vi "AI_StreamingAI_MultipleChannels v6.vi"() -> ()   [LabVIEW 2013]
uses:
  <vilib>/Platform/TimedLoop/XDataNode/timing_clust.ctl
  <vilib>/Platform/TimedLoop/XDataNode/nitl_modes.ctl
  <vilib>/Platform/TimedLoop/XDataNode/wakeup.ctl
  <userlib>/DAQNavi Polymorphic VI/create/DAQNavi Create Channel(AI-Voltage).vi
  <userlib>/DAQNavi Polymorphic VI/configure/timing/DAQNavi Timing(Convert Clock).vi
  <userlib>/DAQNavi Polymorphic VI/configure/DAQNavi Get Property/AI/DAQNaviGet_AI_ConvertClock_Rate.vi
  <userlib>/DAQNavi Polymorphic VI/read/DAQNavi Read (Analog 1D Wfm NChan NSamp).vi
  <vilib>/platform/TimedLoop/XDataNode/XDataNode.xnode
  <vilib>/Platform/TimedLoop/XDataNode/XDNodeRunTimeDep.lvlib
panel:
  out "loop time":dbl format="%.6g"
  in  "Read AtoD":bool
  in  "DO":bool[](array[boolean])
  out "Task5":i32
  out "Test":timestamp
  out "Start":timestamp
  out "loops":bool
  out "error out":errorcluster
  out "Waveform Graph":waveform(dbl)[](graph)
  out "value range":string="+/- 5 V" caption="property value"
  out "physical channels":string="DemoDevice,BID#0/ai0:1" caption="property value"
  in  "Samples":u32=1000
  in  "samples per channel":i32=1024
  out "actual convert rate":dbl
  in  "convert clock rate":dbl=1000.0
  in  "stop":bool
  # "Please modify physical channels and value range in Channel Parameters\nthrough DAQNavi Property Assistant VI  in block diagram."
  # "Channel Parameters"
  # "Timing Parameters"
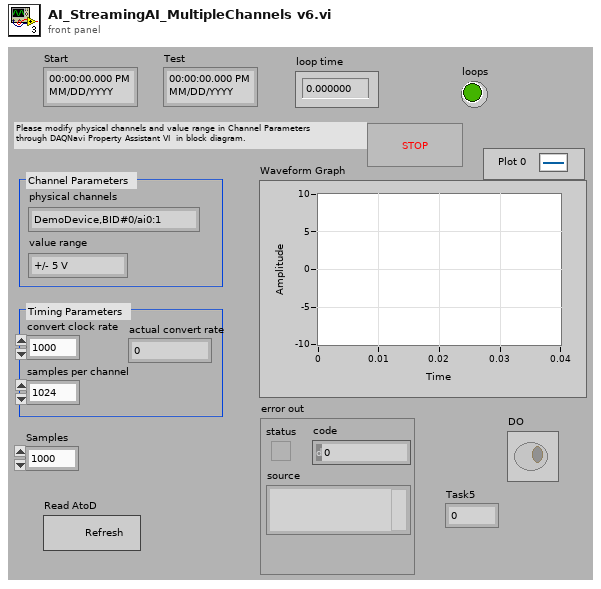
[diagram p1: front panel]
types:
  T1 = typedef "XDNodeRunTimeDep.lvlib/timing_clust.ctl" = cluster{"Expected End [f-1]":u64, "Actual End [f-1]":u64, "Finished Late? [f-1]":bool, "Expected End [i-1]":u64, "Actual End [i-1]":u64, "Finished Late? [i-1]":bool, "Expected Start [i]":u64, "Actual Start [i]":u64, "Expected Start [f]":u64, "Actual Start [f]":u64, "Source Name":string, "Structure Name":string, "Period":i64, "Deadline":i64, "Offset":i64, "Start":i64, "Priority":i32, "Timeout":i32, "Mode":T2, "Wakeup Reason":T3, "Error":errorcluster, "Source Type":string, "Secondary Source Type":string, "Global End Time":u64, "Global Start Time":u64, "Frame Duration":u64, "Iteration Duration":u64, "Assigned CPU":i32, "I/O Scan Engine Mode":u32}
  T2 = typedef "XDNodeRunTimeDep.lvlib/nitl_modes.ctl" = enum32{"No Change", "Process missed periods, maintain original phase", "Discard missed periods, maintain original phase", "Process missed periods, ignore original phase", "Discard missed periods, ignore original phase"}
  T3 = typedef "XDNodeRunTimeDep.lvlib/wakeup.ctl" = enum32{"Normal", "Aborted", "Asynchronous wakeup", "Timing source error", "Timed loop error", "Timeout"}
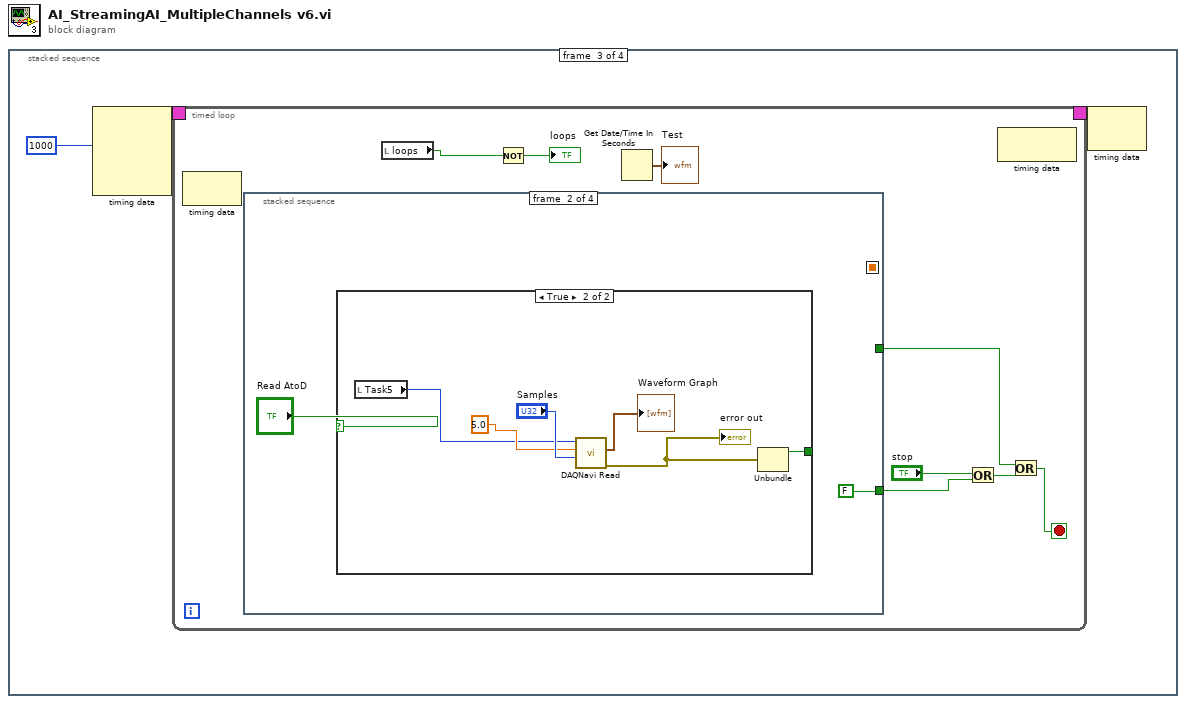
[diagram p0: block diagram]
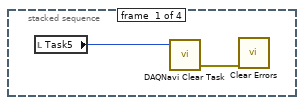
[diagram p2: hidden frame]
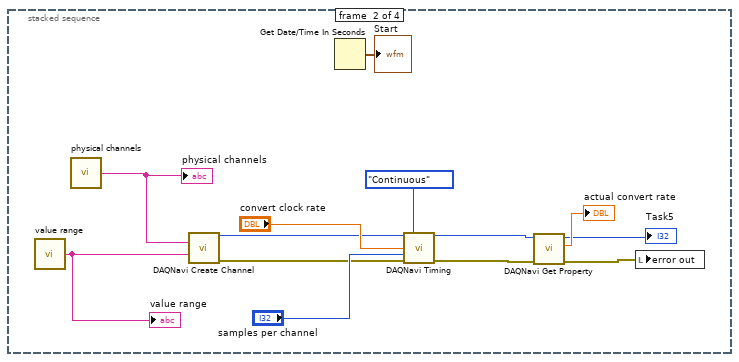
[diagram p3: hidden frame]
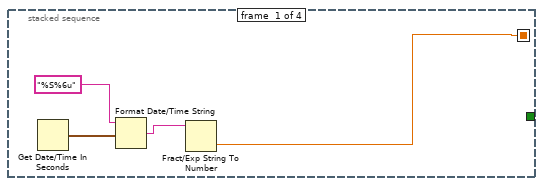
[diagram p4: hidden frame]
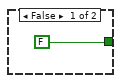
[diagram p5: hidden frame]
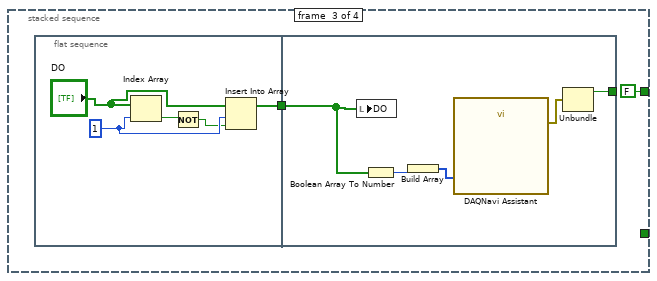
[diagram p6: hidden frame]
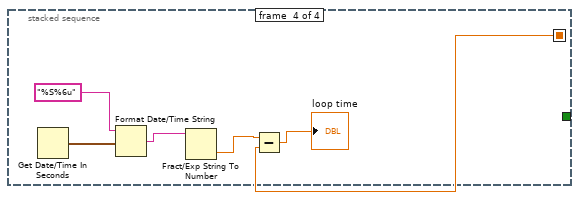
[diagram p7: hidden frame]
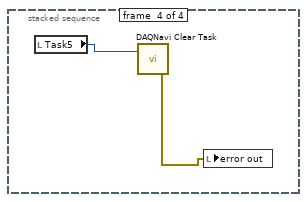
[diagram p8: hidden frame]
diagram:
  n1 = stacked-sequence {
    frame #0 {
      n2 = local read "Task5"() -> (w2:i32)
      n3 = call <userlib>:"DAQNavi Clear Task.vi"("task in"=w2) -> ("error out"=w1:errorcluster)  [unwired: 2 in]
      n4 = call <vilib>:"Clear Errors.vi"("error in (no error)"=w1) -> ()  [unwired: 6 in, 1 out]
    }
    frame #1 {
      n5 = call "value range"() -> ("property value"=w14:string)  [unwired: 1 out]
      "value range" <- w14
      n6 = call "physical channels"() -> ("property value"=w13:string)  [unwired: 1 out]
      "physical channels" <- w13
      n7 = call-poly <userlib>:"DAQNavi Create Channel.vi"("physical channels"=w13, "value range"=w14) -> ("task out"=w5:i32, "error out"=w6:errorcluster)  [unwired: 3 in, 9 out]
      n8 = Get Date/Time In Seconds() -> (seconds since 1Jan1904=→"Start":timestamp)
      n9 = call-poly <userlib>:"DAQNavi Timing.vi"("task in"=w5, "sample mode"=enum16{"Finite", "Continuous"}."Continuous", "rate"="convert clock rate", "samples per channel"="samples per channel", "error in (no error)"=w6) -> ("task out"=w9:i32, "error out"=w10:errorcluster)  [unwired: 1 in, 8 out]
      n10 = call-poly <userlib>:"DAQNavi Get Property.vi"("error in (no error)"=w10, "task in"=w9) -> ("error out"=w4:errorcluster, "rate"=→"actual convert rate":dbl, "task out"=→"Task5":i32)  [unwired: 7 out]
      n11 = local write "error out"(w4) -> ()
    }
    frame #2 {
      n12 = node-c288(1000) -> (w18:T1)  [unwired: 3 in]
      n13 = timed-loop {
        timing: w18 -> [_]
        timing-out: [_] -> w17
        stop <- w23 stop-if-true
        n14 = node-c288() -> ()  [unwired: 1 in, 1 out]
        n15 = stacked-sequence {
          seq-local: [w27 _ _ _] -> [_ _ _ w52]
          tunnel: [_ FALSE _ _] -> w21
          tunnel: [_ _ FALSE _] -> w19
          frame #0 {
            n16 = Get Date/Time In Seconds() -> (seconds since 1Jan1904=w29:timestamp)
            n17 = Format Date/Time String(time format string (%c)="%S%6u", seconds (now)=w29) -> (date/time string=w28:string)  [unwired: 1 in]
            n18 = Fract/Exp String To Number(string=w28) -> (number=w27:dbl)  [unwired: 3 in, 1 out]
          }
          frame #1 {
            n19 = case shown="True" "Read AtoD" {
              tunnel: [FALSE w35] -> _
              frame False {
              }
              frame True {
                n20 = local read "Task5"() -> (w34:i32)
                n21 = call-poly <userlib>:"DAQNavi Read.vi"("number of samples per channel to read"="Samples", "timeout"=5.0, "task in"=w34) -> ("error out"=w36:errorcluster, "data"=→"Waveform Graph":waveform(dbl)[])  [unwired: 1 in, 6 out]
                "error out" <- w36
                n22 = Unbundle(w36) -> ("status"=w35:bool)  [unwired: 2 out]
              }
            }
          }
          frame #2 {
            n23 = flat-sequence {
              tunnel: [w42] -> w41
              tunnel: w41 -> [w50]
              tunnel: [w49] -> _
              frame #0 {
                w46 = 1
                n24 = Index Array(array="DO", index=w46) -> (element=w44:bool)
                n25 = Not(x=w44) -> (.not. x?=w45:bool)
                n26 = Insert Into Array(array="DO", index=w46, new element=w45) -> (w42:bool[])
              }
              frame #1 {
                n27 = local write "DO"(w50) -> ()
                n28 = Boolean Array To Number(Boolean array=w50) -> (number=w51:u32)
                n29 = Build Array(w51) -> (w48:u32[])
                n30 = call "DAQNavi Assistant"("dataIn(U8Array)"=w48) -> ("error out"=w47:errorcluster)  [unwired: 26 in]
                n31 = Unbundle(w47) -> ("status"=w49:bool)  [unwired: 2 out]
              }
            }
          }
          frame #3 {
            n32 = Get Date/Time In Seconds() -> (seconds since 1Jan1904=w56:timestamp)
            n33 = Format Date/Time String(time format string (%c)="%S%6u", seconds (now)=w56) -> (date/time string=w55:string)  [unwired: 1 in]
            n34 = Fract/Exp String To Number(string=w55) -> (number=w54:dbl)  [unwired: 3 in, 1 out]
            n35 = Subtract(x=w54, y=w52) -> (x-y=→"loop time":dbl)
          }
        }
        n36 = local read "loops"() -> (w25:bool)
        n37 = Not(x=w25) -> (.not. x?=→"loops":bool)
        n38 = Get Date/Time In Seconds() -> (seconds since 1Jan1904=→"Test":timestamp)
        n39 = Or(x="stop", y=w21) -> (x .or. y?=w20:bool)
        n40 = node-c288() -> ()  [unwired: 1 in, 1 out]
        n41 = Or(x=w19, y=w20) -> (x .or. y?=w23:bool)
      }
      n42 = node-c288(w17) -> ()  [unwired: 1 out]
    }
    frame #3 {
      n43 = local read "Task5"() -> (w64:i32)
      n44 = call <userlib>:"DAQNavi Clear Task.vi"("task in"=w64) -> ("error out"=w65:errorcluster)  [unwired: 1 in, 1 out]
      n45 = local write "error out"(w65) -> ()
    }
  }
